vi "Init Control.vi"(5 "Group":refnum<class "Group.lvclass">, 7 "VolatusAPI":refnum<class "VolatusAPI.lvclass">, 8 "error in (no error)":errorcluster, 9 "Control MsgQ":refnum<class "MessageQ.lvclass">, 10 "Config Element":refnum<class "Config Element.lvclass">, 11 "LatchedValve in":refnum<class "LatchedValve.lvclass">) -> (0 "error out":errorcluster, 3 "LatchedValve out":refnum<class "LatchedValve.lvclass">)   [LabVIEW 2020, in "VolatusControl.lvlib" / "LatchedValve.lvclass"]
uses:
  LatchedValve.lvclass
  lv-cdm/CDM-Config/Config Element/Config Element.lvclass
  Volatus/VolatusAPI/VolatusAPI.lvclass
  Volatus/MessageQ/MessageQ.lvclass
  LatchedValve.lvclass/LatchedValve.ctl
  lv-cdm/CDM-Config/Config Filter/Config Lookup.lvclass
  lv-vecto/Vecto/GroupAbstract/GroupAbstract.lvclass
  lv-vecto/Vecto/Group/Group.lvclass
  C:/dev/lv20CE/relink/lv-vecto/Vecto/GroupAbstract/GroupAbstract.lvclass
  C:/dev/lv20CE/relink/lv-vecto/Vecto/Group/Group.lvclass
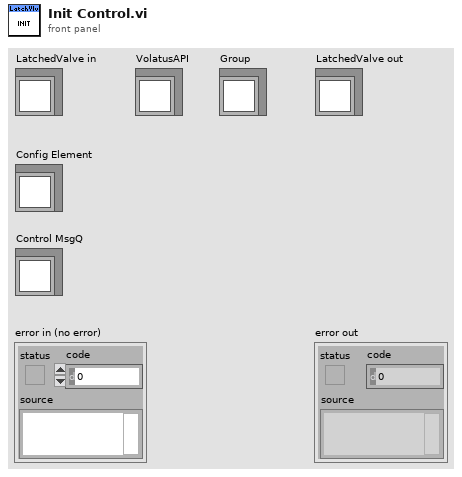
[diagram p1: front panel]
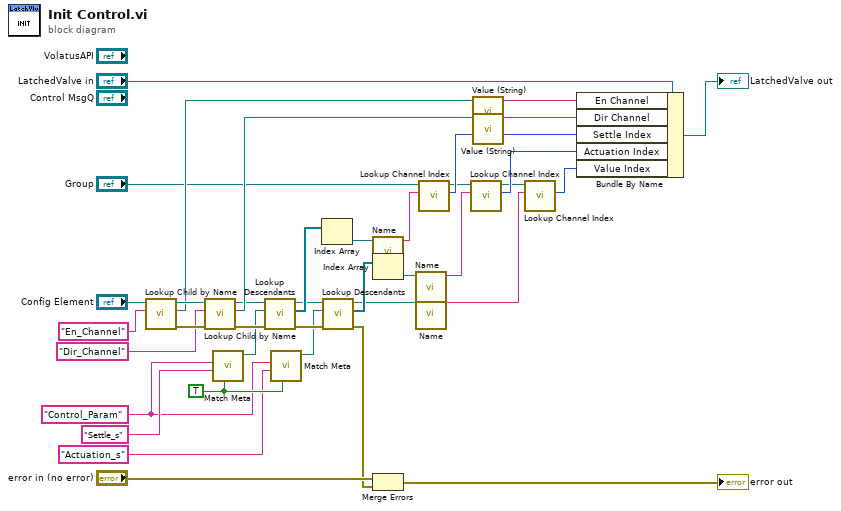
[diagram p0: block diagram]
diagram:
  w19 = TRUE ("Exact Value (F)")
  w18 = "Control_Param" ("Name")
  n1 = call "Lookup Child by Name.vi"("Name"="En_Channel", "Config Element in"="Config Element") -> ("error out"=w36:errorcluster, "Child"=w29:refnum<class "Config Element.lvclass">, "Config Element out"=w30:refnum<class "Config Element.lvclass">)  [unwired: 6 in, 1 out]
  n2 = call "Lookup Child by Name.vi"("error in (no error)"=w36, "Name"="Dir_Channel", "Config Element in"=w30) -> ("error out"=w37:errorcluster, "Child"=w28:refnum<class "Config Element.lvclass">, "Config Element out"=w22:refnum<class "Config Element.lvclass">)  [unwired: 5 in, 1 out]
  n3 = call "Match Meta.vi"("Exact Value (F)"=w19, "Value (Any)"="Settle_s" ("Name"), "Name"=w18) -> ("Config Lookup out"=w23:refnum<class "Config Lookup.lvclass">)  [unwired: 7 in, 1 out]
  n4 = call "Lookup Descendants.vi"("error in (no error)"=w37, "Lookup"=w23, "Config Element in"=w22) -> ("error out"=w38:errorcluster, "Descendants"=w16:refnum<class "Config Element.lvclass">[], "Config Element out"=w14:refnum<class "Config Element.lvclass">)  [unwired: 6 in]
  n5 = call "Match Meta.vi"("Exact Value (F)"=w19, "Value (Any)"="Actuation_s" ("Name"), "Name"=w18) -> ("Config Lookup out"=w20:refnum<class "Config Lookup.lvclass">)  [unwired: 7 in, 1 out]
  n6 = Index Array(array=w16) -> (element=w12:refnum<class "Config Element.lvclass">)  [unwired: 1 in]
  n7 = call "Lookup Descendants.vi"("error in (no error)"=w38, "Lookup"=w20, "Config Element in"=w14) -> ("error out"=w13:errorcluster, "Descendants"=w15:refnum<class "Config Element.lvclass">[], "Config Element out"=w3:refnum<class "Config Element.lvclass">)  [unwired: 6 in]
  n8 = call "Name.vi"("Config Element in"=w12) -> ("Name"=w9:string)  [unwired: 9 in, 1 out]
  n9 = Index Array(array=w15) -> (element=w11:refnum<class "Config Element.lvclass">)  [unwired: 1 in]
  n10 = Merge Errors("error in (no error)", w13) -> (→"error out":errorcluster)
  n11 = call "Name.vi"("Config Element in"=w11) -> ("Name"=w7:string)  [unwired: 9 in, 1 out]
  n12 = call "Name.vi"("Config Element in"=w3) -> ("Name"=w2:string)  [unwired: 9 in, 1 out]
  n13 = call "Lookup Channel Index.vi"("Channel Name"=w9, "GroupAbstract in"="Group") -> ("Index"=w8:i32, "GroupAbstract out"=w6:refnum<class "Group.lvclass">)  [unwired: 7 in, 1 out]
  n14 = call "Lookup Channel Index.vi"("Channel Name"=w7, "GroupAbstract in"=w6) -> ("Index"=w5:i32, "GroupAbstract out"=w4:refnum<class "Group.lvclass">)  [unwired: 7 in, 1 out]
  n15 = call "Value (String).vi"("Config Element in"=w29) -> ("String Value"=w27:string)  [unwired: 9 in, 1 out]
  n16 = call "Value (String).vi"("Config Element in"=w28) -> ("String Value"=w26:string)  [unwired: 9 in, 1 out]
  n17 = call "Lookup Channel Index.vi"("Channel Name"=w2, "GroupAbstract in"=w4) -> ("Index"=w1:i32)  [unwired: 7 in, 2 out]
  n18 = Bundle By Name(cluster="LatchedValve in", "En Channel"=w27, "Dir Channel"=w26, "Settle Index"=w8, "Actuation Index"=w5, "Value Index"=w1) -> (→"LatchedValve out":refnum<class "LatchedValve.lvclass">)
